vi "Test-Light.vi"() -> ()   [LabVIEW 2009]
uses:
  Clients/H5F-File/H5F_ACC.ctl
panel:
  in  "Array":i32[][](array[numeric])=[[0, 0, 0, 0, 0], [0, 0, 0, 0, 1]]
  in  "filename":path
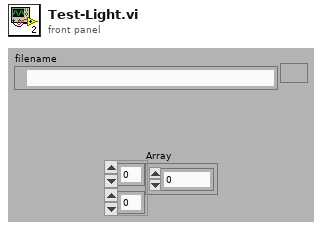
[diagram p1: front panel]
types:
  T1 = typedef "H5F_ACC.ctl" = enum16{"RDONLY", "RDWR", "TRUNC", "EXCL", "DEBUG", "CREAT"}
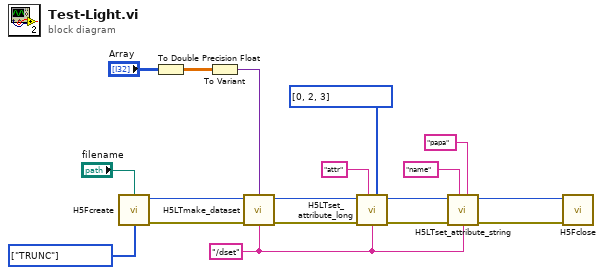
[diagram p0: block diagram]
diagram:
  w2 = "/dset" ("name")
  w12 = T1[] [enum."TRUNC"] items=["RDONLY", "RDWR", "TRUNC", "EXCL", "DEBUG", "CREAT"] ("flags")
  n1 = call "H5Fcreate.vi"("filename"="filename", "flags"=w12) -> ("file_id"=w4:i32, "error out"=w14:errorcluster)  [unwired: 6 in]
  n2 = To Double Precision Float(number="Array") -> (double precision float=w10:dbl[][])
  n3 = To Variant(anything=w10) -> (Variant=w11:variant)
  n4 = call "H5LTmake_dataset.vi"("Array"=w11, "loc_id"=w4, "name"=w2, "error in (no error)"=w14) -> ("error out"=w9:errorcluster)  [unwired: 5 in]
  n5 = call "H5LTset_attribute_long.vi"("error in (no error)"=w9, "name"=w2, "loc_id"=w4, "attr_name"="attr", "buffer"=i32[] [0, 2, 3]) -> ("error out"=w6:errorcluster)  [unwired: 5 in]
  n6 = call "H5LTset_attribute_string.vi"("error in (no error)"=w6, "name"=w2, "loc_id"=w4, "attr_name"="name", "buffer"="papa") -> ("error out"=w5:errorcluster)  [unwired: 5 in]
  n7 = call "H5Fclose.vi"("error in (no error)"=w5, "file_id"=w4) -> ()  [unwired: 8 in, 2 out]
